vi "GA Buf Delay.vi"(7 "segNum":i32, 8 "error in (no error)":errorcluster caption="错误输入（无错误）", 9 "FifoIndex":i16, 10 "ulDelayTime":u32, 11 "nCrdNum":i16) -> (0 "error out":errorcluster caption="错误输出", 3 "function return":i32)   [LabVIEW 2015, in "GAS.lvlib"]
doc: "extern \"C\" __declspec(dllimport) int GA_BufDelay(short nCrdNum,unsigned long ulDelayTime,short FifoIndex=0,long segNum = 0);"
uses:
  <userlib>/BP_GAS/GAS.lvlib
  <userlib>/BP_GAS/GAS.dll
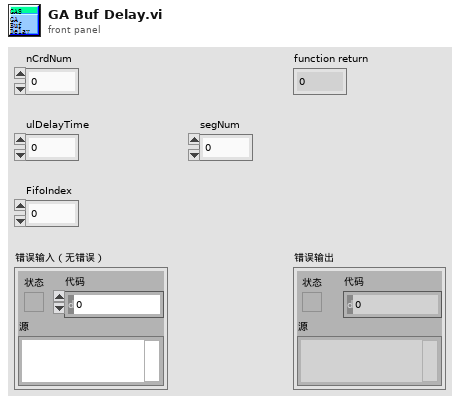
[diagram p1: front panel]
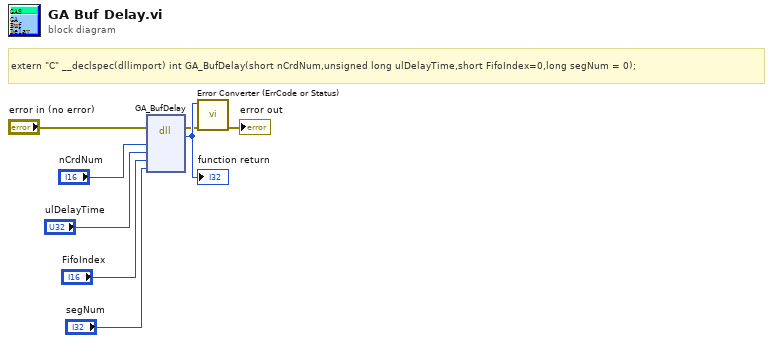
[diagram p0: block diagram]
diagram:
  # "extern \"C\" __declspec(dllimport) int GA_BufDelay(short nCrdNum,unsigned long ulDelayTime,short FifoIndex=0,long segNum = 0);"
  n1 = dll-call lib="E:/Program Files (x86)/National Instruments/LabVIEW 2015/user.lib/BP_GAS/GAS.*" fn="GA_BufDelay"(error in="error in (no error)", "nCrdNum"="nCrdNum", "ulDelayTime"="ulDelayTime", "FifoIndex"="FifoIndex", "segNum"="segNum") -> (error out=w2:errorcluster, w8:i32)  [unwired: 6 in, 1 out]
  "function return" <- w8
  n2 = call "Error Converter (ErrCode or Status).vi"("error in (no error)"=w2, "error code"=w8) -> ("error out"=→"error out":errorcluster)  [unwired: 9 in]
